vi "Get Multi.vi"(0 "Display State In":T30, 5 "Value In":T1={"Waveform"={"Type"=enum."Tone", "Tone"={"Frequency (kHz)"=0.0, "Phase (cycles)"=0.0, "Random phase"=FALSE}, "Pulse Train"={"Pulse width (us)"=0.0, "Pulse rate (Hz)"=0.0, "Gap (ms)"=0.0, "Polarity"=enum."POS", "PT State"={"Template"=[], "Nperiod"=0, "Index"=0, "Pulse Rate (Hz)"=0.0, "Phase (cycles)"=0.0, "Noff"=0}, "Asynch"=FALSE}, "Noise"={"Properties"={"InvFilt"=FALSE, "Aweight"=FALSE, "Seed"=0, "Tokens"=0, "Brickwall"=FALSE}, "Data"={"TokenNum"=0}}, "File"={"Filename"=path "", "Signal"=[], "Channel"=0, "stream"=FALSE, "offset"=0, "nreps"=0, "loops"=0, "Randomize"=FALSE, "order"=[], "Seed"=0, "Tokens"=0}, "FMSweep"={"Rate (oct/s)"=0.0, "Fmin (Hz)"=0.0, "Fmax (Hz)"=0.0, "Ramp (ms)"=0.0, "Linear"=FALSE}, "Chirp Train"={"Params"={"Fmin (kHz)"=4.0, "Fmax (kHz)"=64.0, "Compensate"=FALSE, "Duration (ms)"=2.0}, "Data"={"WF"=[]}}, "Complex Tone"={"Params"={"F0 (Hz)"=0.0, "Band"={"Flow (Hz)"=0.0, "Fhigh (Hz)"=0.0}, "Phase"=enum."Cosine", "Min F0 (Hz)"=0.0, "Max F0 (Hz)"=0.0, "ContinRandPhase"=FALSE, "Max peak factor"=inf, "Max mod depth"=2.0, "MinHarmNum"=0, "MaxHarmNum"=0, "Level Mode"=enum."per component", "% jitter"=0.0}, "Data"={"Ncomp"=0, "MinHarm"=0, "Phase"=[], "Amplitude"=[], "Npts/frame"=0, "Last F0"=0.0, "Fmin"=0.0, "Fmax"=0.0, "Lslope"=0.0, "randphase"=FALSE, "overall rms"=FALSE, "fmult"=[], "jittered"=FALSE}}, "FM"={"Carrier (kHz)"=0.0, "ModRate (Hz)"=0.0, "Depth (Hz)"=0.0, "Phase (cycles)"=0.0}, "Vowel"={"Freqs"="", "Set level"=enum."Total", "Freq"=[], "weights"=[]}, "Ramp"={"Duration (ms)"=0.0}}, "Filter"={"Type"=enum."Lowpass", "CF (kHz)"=0.0, "BW (kHz)"=0.0, "Cascade"=FALSE, "Quadrature"=FALSE, "Scale Factor"=0.0, "Stages"=[], "Class"=enum."Elliptic", "Order"=0, "BWUnits"=enum."Linear"}, "Burst"={"Active"=FALSE, "Delay (ms)"=0.0, "Duration (ms)"=0.0, "Ramp (ms)"=0.0, "Rate (Hz)"=0.0, "Trepeat (ms)"=0.0, "Repeat"=FALSE}, "Level"={"Level"=0.0, "Units"=enum."dB atten", "Max"=0.0, "Data"={"Multiplier"=0.0, "Cal File"=path "", "Cal"={"Freq (Hz)"=[], "Mag (dB SPL)"=[], "Phase (deg)"=[]}, "audiogram"=path ""}}, "Name"="", "Advanced"={"AltPol"=FALSE, "Var"="", "Expr"=""}, "SAM"={"Active"=FALSE, "Frequency (Hz)"=0.0, "Depth"=0.0, "Init Phase (cycles)"=0.0, "phase (degrees)"=0.0, "Asynch"=FALSE}, "Destination"={"Name"="", "Num"=0}} {"Filter"."Stages"."IIR Filter"."Forward Coefficients" format="%.4f"; "Filter"."Stages"."IIR Filter"."Reverse Coefficients" format="%.4f"}, 9 "Container State":T37, 11 "error in (no error)":errorcluster) -> (4 "Display State Out":T30, 6 "Value Out":T1={"Waveform"={"Type"=enum."Tone", "Tone"={"Frequency (kHz)"=0.0, "Phase (cycles)"=0.0, "Random phase"=FALSE}, "Pulse Train"={"Pulse width (us)"=0.0, "Pulse rate (Hz)"=0.0, "Gap (ms)"=0.0, "Polarity"=enum."POS", "PT State"={"Template"=[], "Nperiod"=0, "Index"=0, "Pulse Rate (Hz)"=0.0, "Phase (cycles)"=0.0, "Noff"=0}, "Asynch"=FALSE}, "Noise"={"Properties"={"InvFilt"=FALSE, "Aweight"=FALSE, "Seed"=0, "Tokens"=0, "Brickwall"=FALSE}, "Data"={"TokenNum"=0}}, "File"={"Filename"=path "", "Signal"=[], "Channel"=0, "stream"=FALSE, "offset"=0, "nreps"=0, "loops"=0, "Randomize"=FALSE, "order"=[], "Seed"=0, "Tokens"=0}, "FMSweep"={"Rate (oct/s)"=0.0, "Fmin (Hz)"=0.0, "Fmax (Hz)"=0.0, "Ramp (ms)"=0.0, "Linear"=FALSE}, "Chirp Train"={"Params"={"Fmin (kHz)"=4.0, "Fmax (kHz)"=64.0, "Compensate"=FALSE, "Duration (ms)"=2.0}, "Data"={"WF"=[]}}, "Complex Tone"={"Params"={"F0 (Hz)"=0.0, "Band"={"Flow (Hz)"=0.0, "Fhigh (Hz)"=0.0}, "Phase"=enum."Cosine", "Min F0 (Hz)"=0.0, "Max F0 (Hz)"=0.0, "ContinRandPhase"=FALSE, "Max peak factor"=inf, "Max mod depth"=2.0, "MinHarmNum"=0, "MaxHarmNum"=0, "Level Mode"=enum."per component", "% jitter"=0.0}, "Data"={"Ncomp"=0, "MinHarm"=0, "Phase"=[], "Amplitude"=[], "Npts/frame"=0, "Last F0"=0.0, "Fmin"=0.0, "Fmax"=0.0, "Lslope"=0.0, "randphase"=FALSE, "overall rms"=FALSE, "fmult"=[], "jittered"=FALSE}}, "FM"={"Carrier (kHz)"=0.0, "ModRate (Hz)"=0.0, "Depth (Hz)"=0.0, "Phase (cycles)"=0.0}, "Vowel"={"Freqs"="", "Set level"=enum."Total", "Freq"=[], "weights"=[]}, "Ramp"={"Duration (ms)"=0.0}}, "Filter"={"Type"=enum."Lowpass", "CF (kHz)"=0.0, "BW (kHz)"=0.0, "Cascade"=FALSE, "Quadrature"=FALSE, "Scale Factor"=0.0, "Stages"=[], "Class"=enum."Elliptic", "Order"=0, "BWUnits"=enum."Linear"}, "Burst"={"Active"=FALSE, "Delay (ms)"=0.0, "Duration (ms)"=0.0, "Ramp (ms)"=0.0, "Rate (Hz)"=0.0, "Trepeat (ms)"=0.0, "Repeat"=FALSE}, "Level"={"Level"=0.0, "Units"=enum."dB atten", "Max"=0.0, "Data"={"Multiplier"=0.0, "Cal File"=path "", "Cal"={"Freq (Hz)"=[], "Mag (dB SPL)"=[], "Phase (deg)"=[]}, "audiogram"=path ""}}, "Name"="", "Advanced"={"AltPol"=FALSE, "Var"="", "Expr"=""}, "SAM"={"Active"=FALSE, "Frequency (Hz)"=0.0, "Depth"=0.0, "Init Phase (cycles)"=0.0, "phase (degrees)"=0.0, "Asynch"=FALSE}, "Destination"={"Name"="", "Num"=0}} {"Filter"."Stages"."IIR Filter"."Forward Coefficients" format="%.4f"; "Filter"."Stages"."IIR Filter"."Reverse Coefficients" format="%.4f"}, 15 "error out":errorcluster)   [LabVIEW 2020, in "Stimulus Channel (G3).xctl"]
uses:
  Stimulus Channel (G3).xctl
  Utility VIs/Controls/KRing/KRing.xctl
  Level (G3)/Level (G3).xctl
  Burst (G3)/Burst (G3).xctl
  Waveform XControls/Waveform (G3)/Waveform (G3).xctl
  <vilib>/_xctls/Container State.ctl
  <vilib>/_xctls/XControlSupport.lvlib
  Level (G3)/Level Units (G3).ctl
  Waveform XControls/Noise (G3)/Noise (G3) - Persistent.ctl
  Waveform XControls/Noise (G3)/Noise (G3).xctl
  Waveform XControls/Waveform (G3)/Waveform (G3) - Persistent.ctl
  Calibration VIs/Endpoint VIs/LV Source/Endpoint-Laterality.ctl
  Calibration VIs/Endpoint VIs/LV Source/Endpoint-Modality.ctl
  Calibration VIs/Endpoint VIs/LV Source/Endpoint-Spec.ctl
  State.ctl
  Filter (G3)/Filter Type.ctl
  Filter (G3)/Filter (G3).xctl
  Filter VIs/Filter-Bandwidth Units.ctl
  Filter (G3)/Filter Data.ctl
  Level (G3)/Level Data.ctl
  Controls/Burst XCtl/Burst Data.ctl
  Controls/Burst XCtl/Burst Control.xctl
  Waveform XControls/Tone (G3)/Tone.Properties.ctl
  Waveform XControls/Tone (G3)/Tone (G3).xctl
  Waveform VIs/Pulse Train VIs/Pulse Polarity.ctl
  Waveform VIs/Pulse Train VIs/PT-Continuous State.ctl
  Waveform VIs/Pulse Train VIs/Pulse Train Params.ctl
  Waveform VIs/Noise VIs/Noise (G3).Properties.ctl
  Waveform VIs/Noise VIs/Noise (G3).Data.ctl
  Waveform VIs/Noise VIs/Noise (G3).ctl
  Waveform VIs/File VIs/StimFile-Params.ctl
  Waveform VIs/FM Sweep VIs/FM Sweep Params.ctl
  Waveform VIs/Chirp Train VIs/Chirp Train Params.ctl
  Waveform VIs/Chirp Train VIs/Chirp Train.ctl
  Waveform VIs/Complex Tone VIs/CT-Phase Enum.ctl
  Waveform VIs/Complex Tone VIs/CT-Params.ctl
  Waveform VIs/Complex Tone VIs/CT-Runtime Data.ctl
  Waveform XControls/FM Tone/Data.ctl
  Waveform XControls/FM Tone/FM Tone.xctl
  Waveform XControls/Waveform (G3)/Waveform Data.ctl
  Advanced Options (G3)/Advanced Options (G3).ctl
  Advanced Options (G3)/Advanced Options (G3).xctl
  Modulation VIs/SAM VIs/SAM Params.ctl
  Typedefs/Destination.ctl
  Full Stimulus Channel Data.ctl
  Burst (G3)/Controls.ctl
  Waveform XControls/Vowel/Vowel.Properties.ctl
  Waveform XControls/Vowel/Vowel.xctl
  Waveform VIs/Waveform Enum (V3).ctl
  Waveform VIs/Ramp VIs/Ramp.Properties.ctl
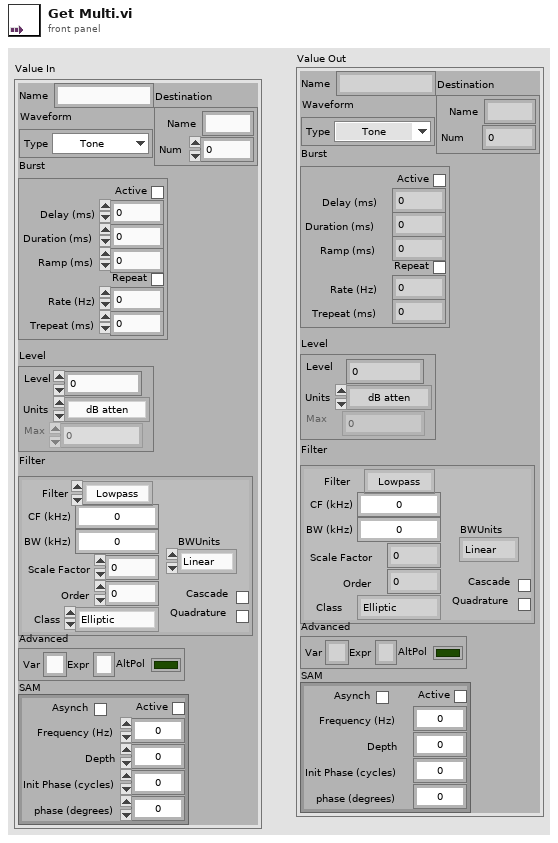
[diagram p1: front panel]
types:
  T1 = typedef "Stimulus Channel (G3).xctl/Full Stimulus Channel Data.ctl" = cluster{"Waveform":T2, "Filter":T21, "Burst":T24, "Level":T25, "Name":string, "Advanced":T27, "SAM":T28, "Destination":T29}
  T2 = typedef "Waveform (G3).xctl/Waveform Data.ctl" = cluster{"Type":T3, "Tone":T4, "Pulse Train":T5, "Noise":T8, "File":T11, "FMSweep":T12, "Chirp Train":T13, "Complex Tone":cluster{"Params":T15, "Data":T17}, "FM":T18, "Vowel":T19, "Ramp":T20}
  T3 = typedef "Waveform Enum (V3).ctl" = enum16{"OFF", "Tone", "Noise", "Pulse Train", "File", "FM Sweep", "Chirp Train", "Complex Tone", "FM Tone", "Vowel", "Ramp"}
  T4 = typedef "Tone (G3).xctl/Tone.Properties.ctl" = cluster{"Frequency (kHz)":dbl, "Phase (cycles)":dbl, "Random phase":bool}
  T5 = typedef "Pulse Train Params.ctl" = cluster{"Pulse width (us)":dbl, "Pulse rate (Hz)":dbl, "Gap (ms)":dbl, "Polarity":T6, "PT State":T7, "Asynch":bool}
  T6 = typedef "Pulse Polarity.ctl" = enum16{"POS", "NEG", "POS-NEG", "NEG-POS"}
  T7 = typedef "PT-Continuous State.ctl" = cluster{"Template":dbl[], "Nperiod":i32, "Index":i32, "Pulse Rate (Hz)":dbl, "Phase (cycles)":dbl, "Noff":i32}
  T8 = typedef "Noise (G3).ctl" = cluster{"Properties":T9, "Data":T10}
  T9 = typedef "Noise (G3).Properties.ctl" = cluster{"InvFilt":bool, "Aweight":bool, "Seed":i32, "Tokens":i32, "Brickwall":bool}
  T10 = typedef "Noise (G3).Data.ctl" = cluster{"TokenNum":i32}
  T11 = typedef "StimFile-Params.ctl" = cluster{"Filename":path, "Signal":dbl[], "Channel":i32, "stream":bool, "offset":i32, "nreps":i32, "loops":i32, "Randomize":bool, "order":i32[], "Seed":i32, "Tokens":i32}
  T12 = typedef "FM Sweep Params.ctl" = cluster{"Rate (oct/s)":dbl, "Fmin (Hz)":dbl, "Fmax (Hz)":dbl, "Ramp (ms)":dbl, "Linear":bool}
  T13 = typedef "Chirp Train.ctl" = cluster{"Params":T14, "Data":cluster{"WF":dbl[]}}
  T14 = typedef "Chirp Train Params.ctl" = cluster{"Fmin (kHz)":dbl, "Fmax (kHz)":dbl, "Compensate":bool, "Duration (ms)":dbl}
  T15 = typedef "CT-Params.ctl" = cluster{"F0 (Hz)":dbl, "Band":cluster{"Flow (Hz)":dbl, "Fhigh (Hz)":dbl}, "Phase":T16, "Min F0 (Hz)":dbl, "Max F0 (Hz)":dbl, "ContinRandPhase":bool, "Max peak factor":dbl, "Max mod depth":dbl, "MinHarmNum":i32, "MaxHarmNum":i32, "Level Mode":enum16{"per component", "overall rms"}, "% jitter":dbl}
  T16 = typedef "CT-Phase Enum.ctl" = enum16{"Cosine", "Random", "Alternating"}
  T17 = typedef "CT-Runtime Data.ctl" = cluster{"Ncomp":i32, "MinHarm":i32, "Phase":dbl[], "Amplitude":dbl[], "Npts/frame":i32, "Last F0":dbl, "Fmin":dbl, "Fmax":dbl, "Lslope":dbl, "randphase":bool, "overall rms":bool, "fmult":dbl[], "jittered":bool}
  T18 = typedef "FM Tone.xctl/Data.ctl" = cluster{"Carrier (kHz)":dbl, "ModRate (Hz)":dbl, "Depth (Hz)":dbl, "Phase (cycles)":dbl}
  T19 = typedef "Vowel.xctl/Vowel.Properties.ctl" = cluster{"Freqs":string, "Set level":enum16{"Total", "Per component"}, "Freq":dbl[], "weights":dbl[]}
  T20 = typedef "Ramp.Properties.ctl" = cluster{"Duration (ms)":dbl}
  T21 = typedef "Filter (G3).xctl/Filter Data.ctl" = cluster{"Type":T22, "CF (kHz)":dbl, "BW (kHz)":dbl, "Cascade":bool, "Quadrature":bool, "Scale Factor":dbl, "Stages":cluster{"IIR Filter":cluster{"filter structure":enum32{"IIR 2nd Order", "IIR 4th Order"}, "Reverse Coefficients":dbl[], "Forward Coefficients":dbl[]}, "State":dbl[]}[], "Class":enum16{"Elliptic", "Butterworth"}, "Order":i32, "BWUnits":T23}
  T22 = typedef "Filter (G3).xctl/Filter Type.ctl" = enum16{"OFF", "Lowpass", "Highpass", "Bandpass", "Bandstop"}
  T23 = typedef "Filter-Bandwidth Units.ctl" = enum16{"Linear", "Octaves", "Min-Max"}
  T24 = typedef "Burst Control.xctl/Burst Data.ctl" = cluster{"Active":bool, "Delay (ms)":dbl, "Duration (ms)":dbl, "Ramp (ms)":dbl, "Rate (Hz)":dbl, "Trepeat (ms)":dbl, "Repeat":bool}
  T25 = typedef "Level (G3).xctl/Level Data.ctl" = cluster{"Level":dbl, "Units":T26, "Max":dbl, "Data":cluster{"Multiplier":dbl, "Cal File":path, "Cal":cluster{"Freq (Hz)":dbl[], "Mag (dB SPL)":dbl[], "Phase (deg)":dbl[]}, "audiogram":path}}
  T26 = typedef "Level (G3).xctl/Level Units (G3).ctl" = enum16{"dB atten", "dB SPL", "dB re 1 Vrms", "dB V/Hz½", "mW", "dB HL", "Volts", "dB mW"}
  T27 = typedef "Advanced Options (G3).xctl/Advanced Options (G3).ctl" = cluster{"AltPol":bool, "Var":string, "Expr":string}
  T28 = typedef "SAM Params.ctl" = cluster{"Active":bool, "Frequency (Hz)":dbl, "Depth":dbl, "Init Phase (cycles)":dbl, "phase (degrees)":dbl, "Asynch":bool}
  T29 = typedef "Destination.ctl" = cluster{"Name":string, "Num":i32}
  T30 = typedef "Stimulus Channel (G3).xctl/State.ctl" = cluster{"Show advanced":bool, "Show rove":bool, "Show name":bool, "Show dest":bool, "Lock dest":bool, "max level":dbl, "LMax Event":refnum<user-event>, "Controls":T31, "Level units":T26[], "Waveforms":T3[], "waveform":T32, "Endpoint Config":T34[], "multi":bool}
  T31 = typedef "Controls.ctl" = cluster{"Waveform":refnum<vi>, "Level":refnum<vi>, "Dest":refnum<vi>, "Gate":refnum<vi>}
  T32 = typedef "Waveform (G3).xctl/Waveform (G3) - Persistent.ctl" = cluster{"noise":T33, "Sort":bool}
  T33 = typedef "Noise (G3).xctl/Noise (G3) - Persistent.ctl" = cluster{"Show Aweight":bool}
  T34 = typedef "Endpoint-Spec.ctl" = cluster{"Name":string, "Modality":T35, "Laterality":T36, "CalFile":path, "Audiogram":path, "reuse cal?":bool}
  T35 = typedef "Endpoint-Modality.ctl" = enum16{"Unspecified", "Acoustic", "Electric", "Optical"}
  T36 = typedef "Endpoint-Laterality.ctl" = enum16{"N/A", "Right", "Left"}
  T37 = typedef "XControlSupport.lvlib/Container State.ctl" = cluster{"Indicator?":bool, "Run Mode?":bool, " Refnum":refnum<vi>}
  T38 = typedef "Burst (G3).xctl/Burst Data.ctl" = cluster{"Active":bool, "Delay (ms)":dbl, "Duration (ms)":dbl, "Ramp (ms)":dbl, "Rate (Hz)":dbl, "Trepeat (ms)":dbl, "Repeat":bool}
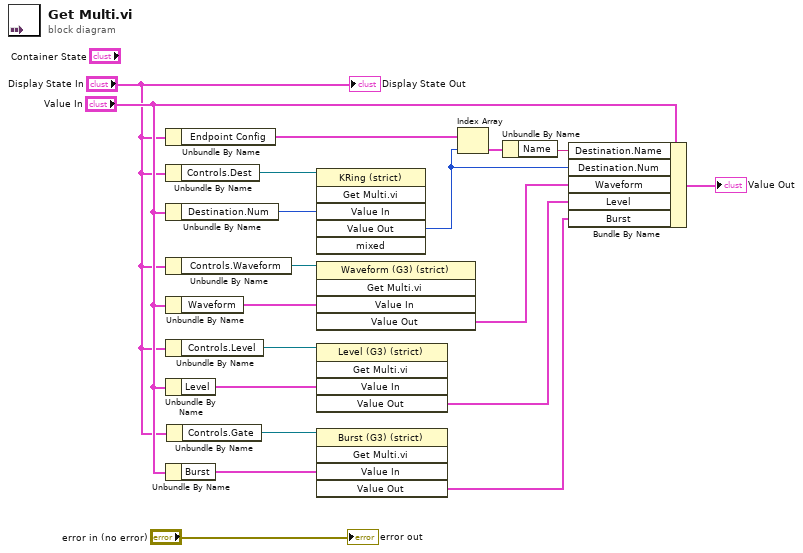
[diagram p0: block diagram]
diagram:
  n1 = Unbundle By Name("Display State In") -> ("Endpoint Config"=w17:T34[])
  n2 = Unbundle By Name("Display State In") -> ("Controls.Dest"=w13:refnum<vi>)
  n3 = Unbundle By Name("Value In") -> ("Destination.Num"=w12:i32)
  n4 = Unbundle By Name("Display State In") -> ("Controls.Waveform"=w2:refnum<vi>)
  n5 = Unbundle By Name("Value In") -> ("Waveform"=w1:T2)
  n6 = Unbundle By Name("Display State In") -> ("Controls.Level"=w10:refnum<vi>)
  n7 = Unbundle By Name("Value In") -> ("Level"=w9:T25)
  n8 = Unbundle By Name("Value In") -> ("Burst"=w6:T24)
  n9 = Unbundle By Name("Display State In") -> ("Controls.Gate"=w7:refnum<vi>)
  n10 = invoke class="KRing (strict)" method="Get Multi.vi"(reference=w13, "Value In"=w12) -> ("Value Out"=w11:i16)  [unwired: 4 in, 5 out]
  n11 = invoke class="Waveform (G3) (strict)" method="Get Multi.vi"(reference=w2, "Value In"=w1) -> ("Value Out"=w14:T2)  [unwired: 3 in, 4 out]
  n12 = invoke class="Level (G3) (strict)" method="Get Multi.vi"(reference=w10, "Value In"=w9) -> ("Value Out"=w8:T25)  [unwired: 3 in, 4 out]
  n13 = invoke class="Burst (G3) (strict)" method="Get Multi.vi"(reference=w7, "Value In"=w6) -> ("Value Out"=w3:T38)  [unwired: 3 in, 4 out]
  n14 = Index Array(array=w17, index=w11) -> (element=w16:T34)
  n15 = Unbundle By Name(w16) -> ("Name"=w15:string)
  n16 = Bundle By Name(cluster="Value In", "Destination.Name"=w15, "Destination.Num"=w11, "Waveform"=w14, "Level"=w8, "Burst"=w3) -> (→"Value Out":T1)
  "Display State Out" <- "Display State In"
  "error out" <- "error in (no error)"
